vi "user process.vi"(8 "error in":errorcluster, 10 "MotionModule runtime in":refnum<class "MotionModule runtime.lvclass">, 11 "Parameters to process":T2) -> (0 "error out":errorcluster, 2 "MotionModule runtime Out":refnum<class "MotionModule runtime.lvclass">, 3 "Results from processing":T1)   [LabVIEW 2017, in "MotionModule runtime.lvclass"]
uses:
  MotionModule runtime.lvclass
  parameter user data.ctl
  result user data.ctl
  MotionModule runtime.lvclass/MotionModule runtime.ctl
  Utilities/StateMachine.ctl
  SoftmotionClass/SoftmotionAxis/SoftmotionAxis.lvclass
  Utilities/Controlword_Commands.ctl
  Utilities/MoveMode.ctl
  Utilities/WordManipulationLibrary.lvlib
  Utilities/Bit Manipulation.lvlib
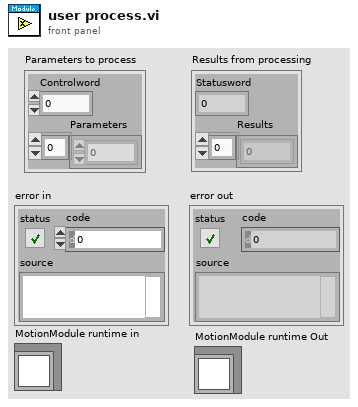
[diagram p1: front panel]
types:
  T1 = typedef "MotionModule runtime.lvclass/result user data.ctl" = cluster{"Statusword":u16, "Results":dbl[]}
  T2 = typedef "MotionModule runtime.lvclass/parameter user data.ctl" = cluster{"Controlword":u16, "Parameters":dbl[]}
  T3 = typedef "WordManipulationLibrary.lvlib/StateMachine.ctl" = enum16{"Start", "Not Ready to Switch On", "Switch On Disabled", "Ready to Switch On", "Switched On", "Operation enable", "Quick Stop Active", "Fault Reaction Active", "Fault"}
  T4 = typedef "WordManipulationLibrary.lvlib/Controlword_Commands.ctl" = enum16{"Shutdown", "Switch On", "Disable Voltage", "Quick Stop", "Disable Op", "Enable Op", "Fault Reset", "Error"}
  T5 = typedef "WordManipulationLibrary.lvlib/MoveMode.ctl" = enum16{"Reserved", "Profile Position Mode", "Velocity Mode", "Profile Velocity Mode", "Profile Torque Mode", "Reserved 2", "Reference Mode", "Interpolated Position Mode", "Skip"}
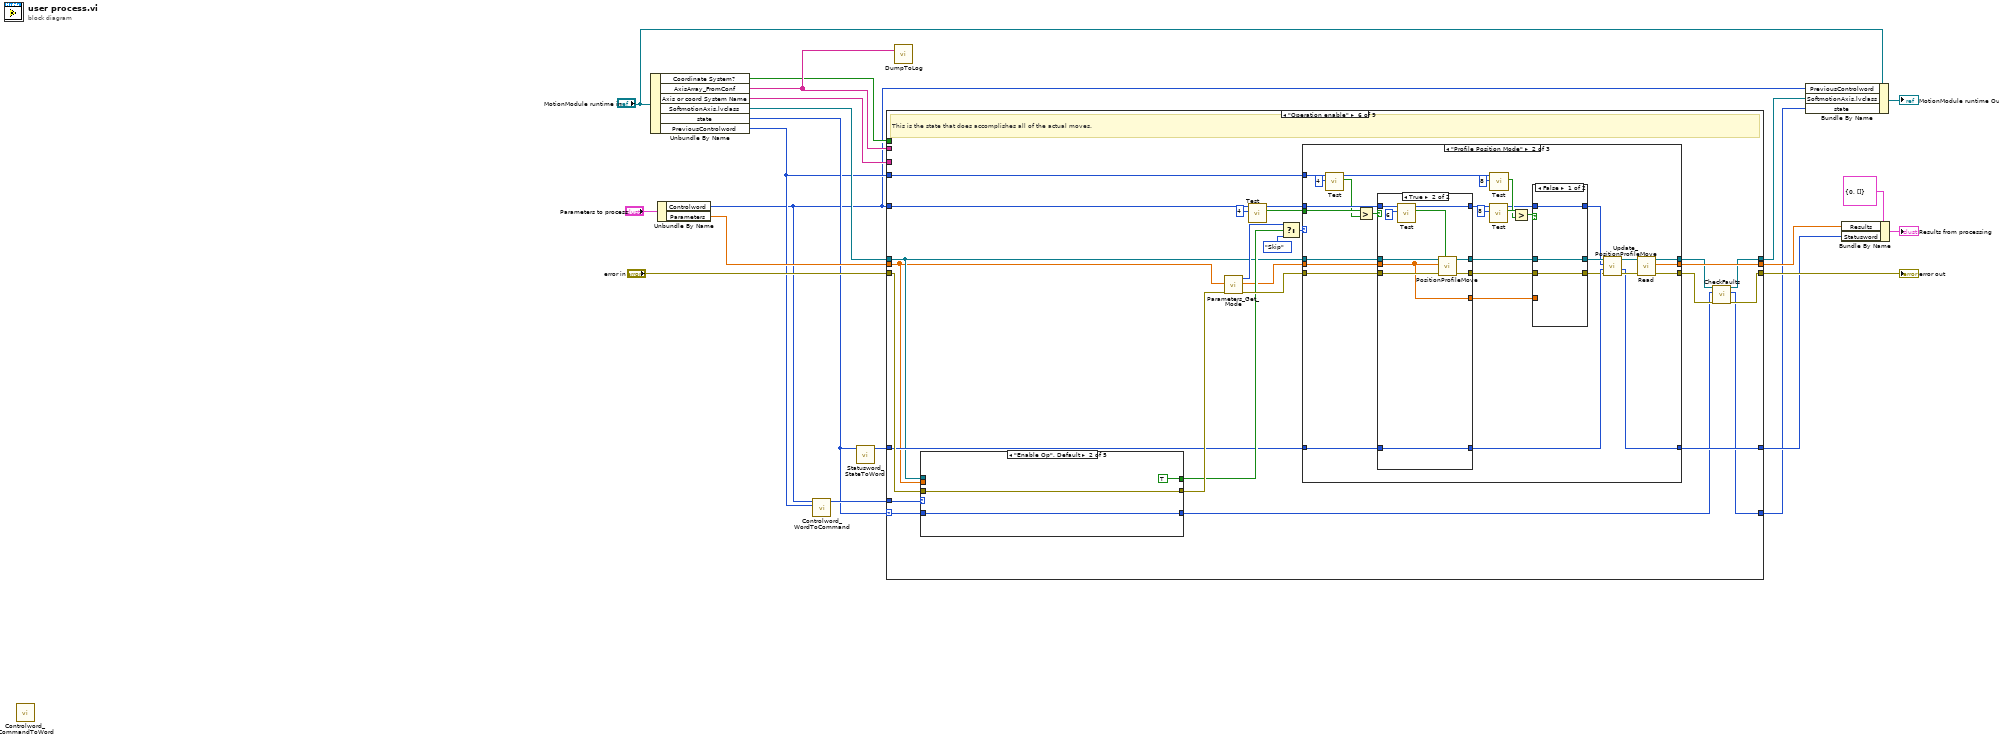
[diagram p0: block diagram]
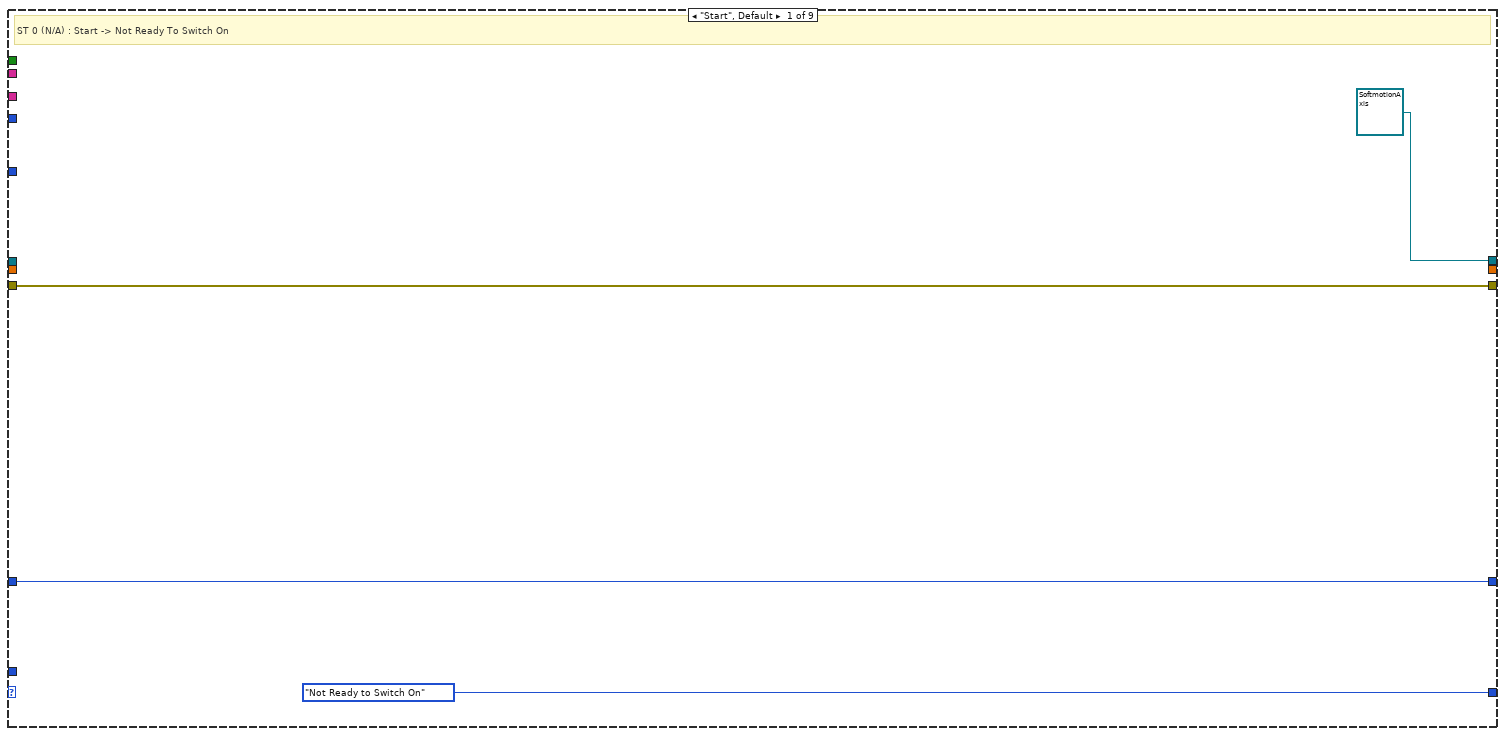
[diagram p2: hidden frame]
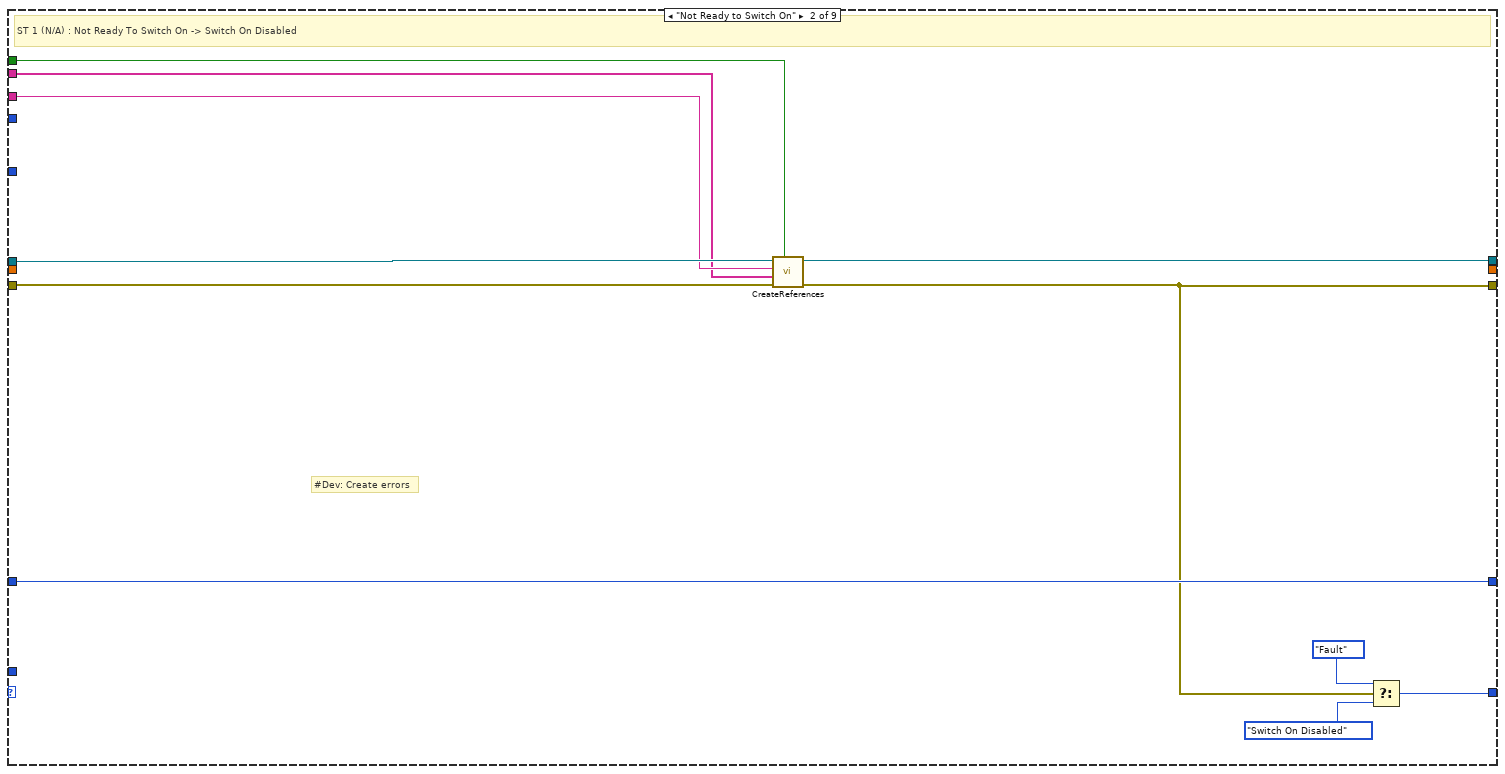
[diagram p3: hidden frame]
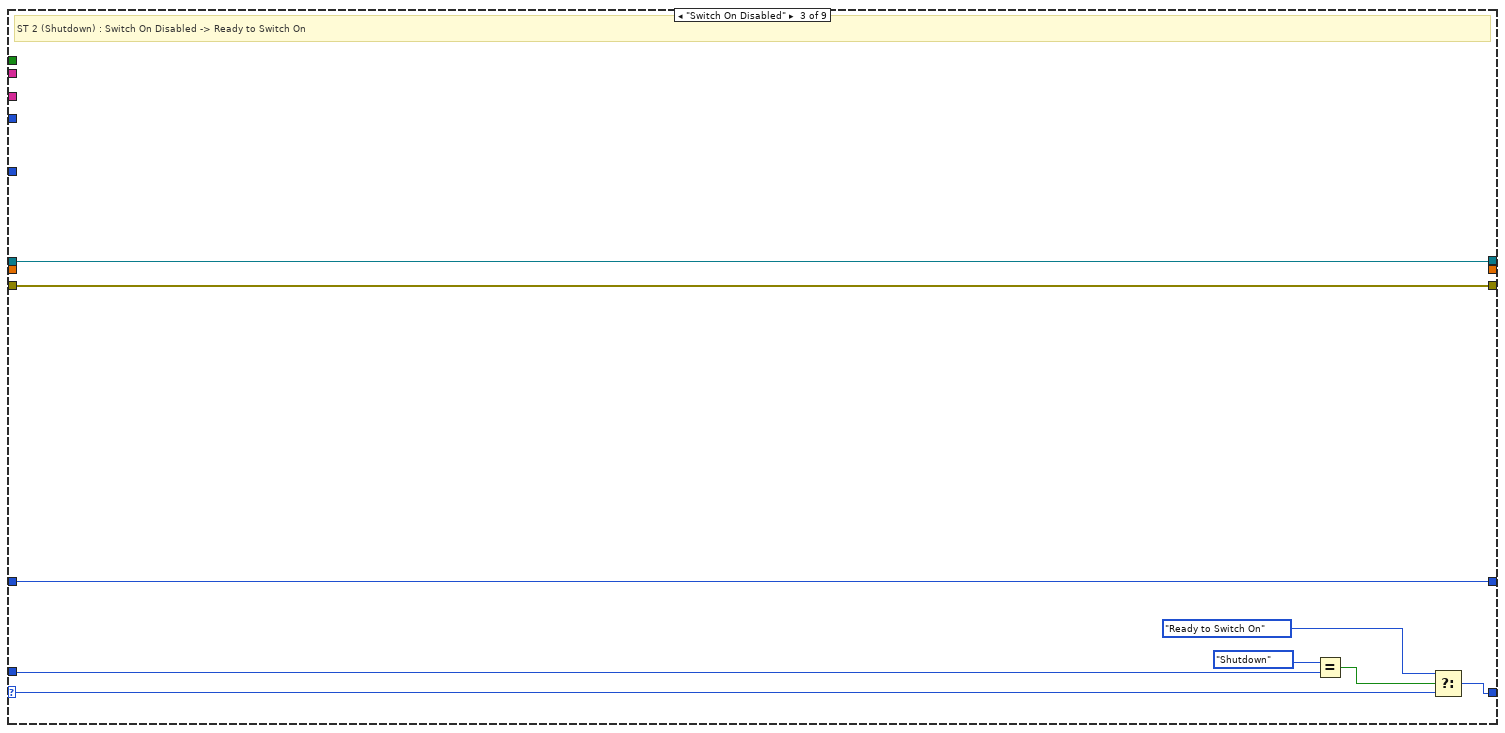
[diagram p4: hidden frame]
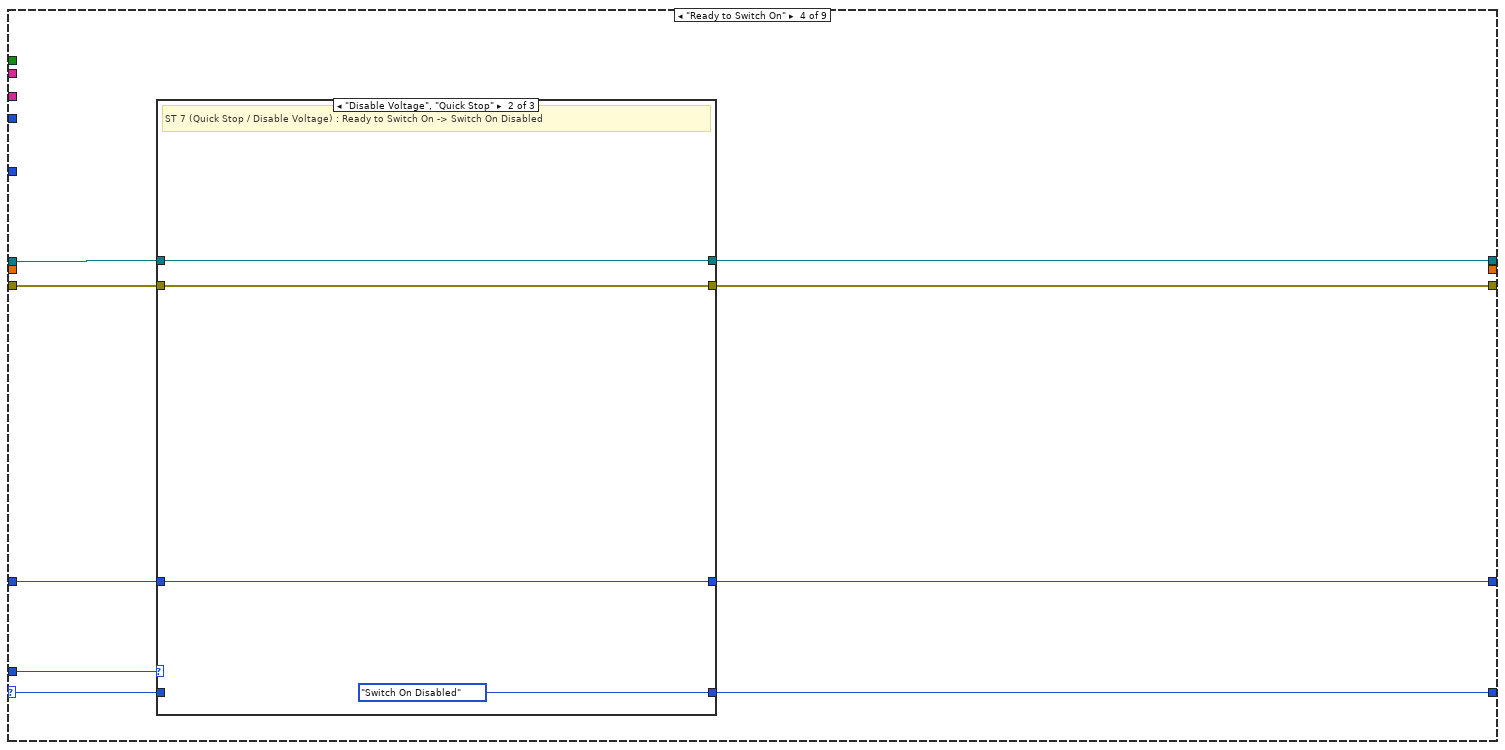
[diagram p5: hidden frame]
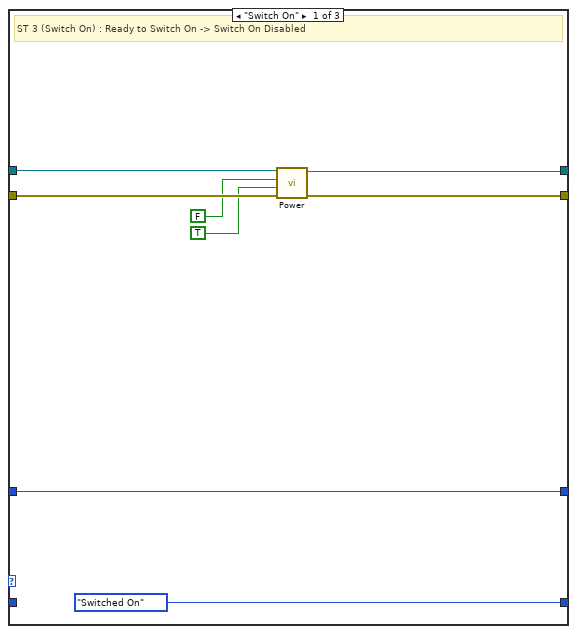
[diagram p6: hidden frame]
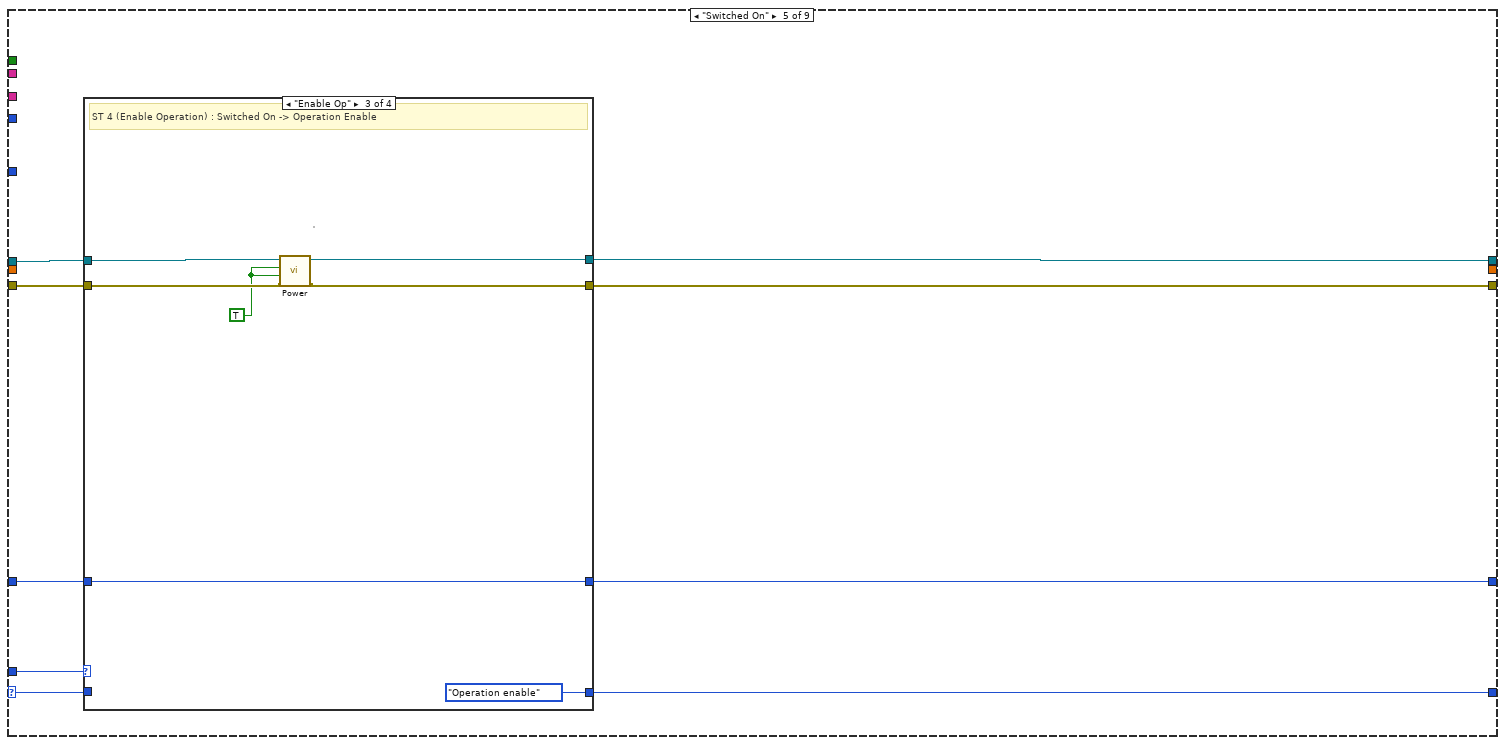
[diagram p8: hidden frame]
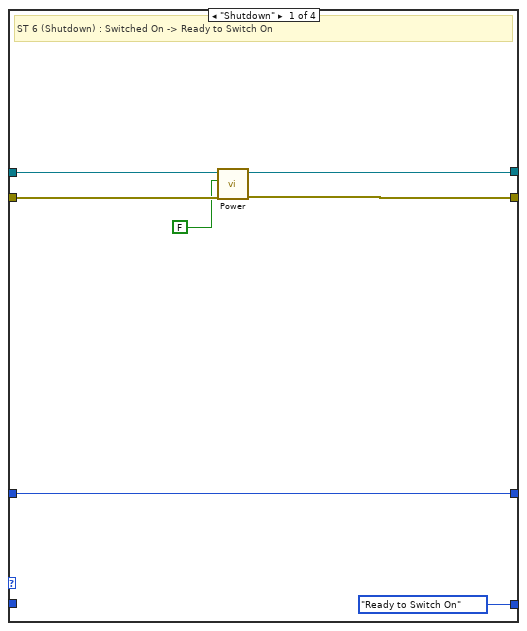
[diagram p9: hidden frame]
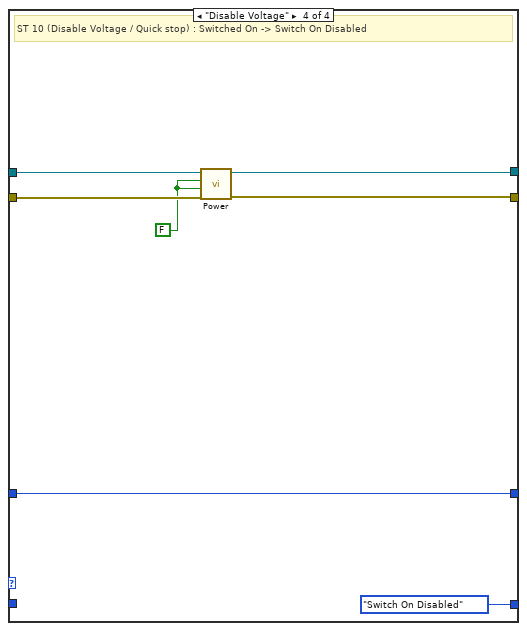
[diagram p11: hidden frame]
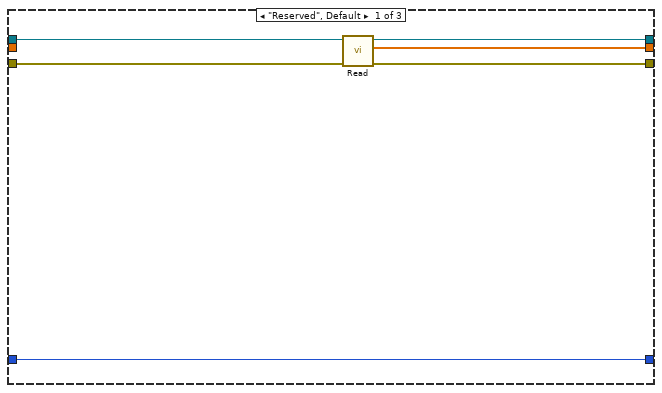
[diagram p12: hidden frame]
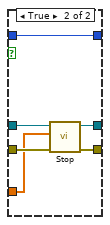
[diagram p13: hidden frame]
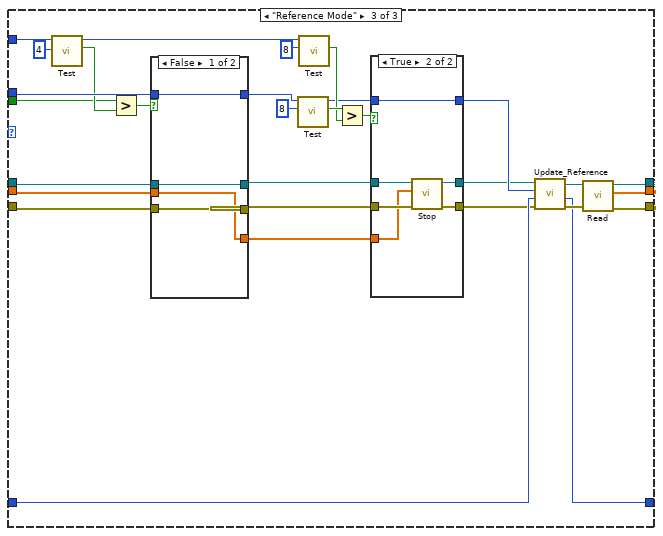
[diagram p15: hidden frame]
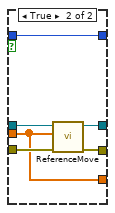
[diagram p17: hidden frame]
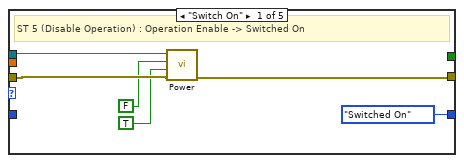
[diagram p18: hidden frame]
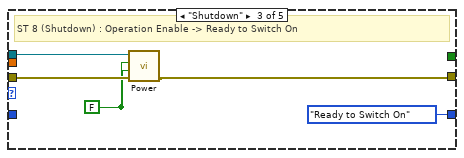
[diagram p19: hidden frame]
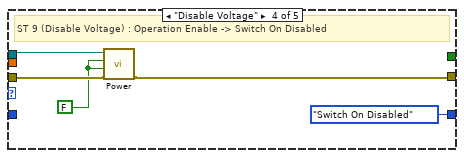
[diagram p20: hidden frame]
diagram:
  n1 = call "Controlword_CommandToWord.vi"() -> ()  [unwired: 11 in, 1 out]
  n2 = Unbundle By Name("MotionModule runtime in") -> ("Coordinate System?"=w2:bool, "AxisArray_FromConf"=w3:string[], "Axis or coord System Name"=w5:string, "SoftmotionAxis.lvclass"=w15:refnum<class "SoftmotionAxis.lvclass">, "state"=w7:T3, "PreviousControlword"=w4:u16)
  n3 = Unbundle By Name("Parameters to process") -> ("Controlword"=w1:u16, "Parameters"=w18:dbl[])
  n4 = call "Controlword_WordToCommand.vi"("Previous Controlword"=w4, "Controlword"=w1) -> ("Device Control Command"=w20:T4)  [unwired: 9 in]
  n5 = call "Statusword_StateToWord.vi"("CurrentStatus"=w7) -> ("StatusWord Out"=w21:u16)  [unwired: 10 in]
  n6 = case shown="\"Operation enable\"" w7 {
    selector: w7 -> [_ _ w41 w53 w78 w129 w267 _ w285]
    tunnel: w20 -> [_ _ w45 w54 w79 w130 w269 _ w286]
    tunnel: [StateMachine."Not Ready to Switch On" w33 w40 w52 w77 w107 w268 StateMachine."Fault" w287] -> w6
    tunnel: [w24 w36 w39 w48 w74 w126 w266 w278 w284] -> w8
    tunnel: w21 -> [w24 w36 w39 w49 w75 w115 w266 w278 w284]
    tunnel: w1 -> [_ _ _ _ _ w128 _ _ _]
    tunnel: w18 -> [_ _ _ _ _ w105 _ _ _]
    tunnel: w5 -> [_ w28 _ _ _ _ _ _ _]
    tunnel: [_ _ _ _ _ w125 _ _ _] -> w9
    tunnel: "error in" -> [w23 w32 w38 w51 w76 w121 _ w275 w283]
    tunnel: [w23 w29 w38 w50 w73 w111 _ w274 w282] -> w16
    tunnel: w15 -> [_ w31 w37 w47 w72 w113 w265 w277 w281]
    tunnel: [refnum<class "SoftmotionAxis.lvclass"> refnum ("SoftmotionAxis.lvclass") w30 w37 w46 w71 w109 w265 w276 w280] -> w13
    tunnel: w4 -> [_ _ _ _ _ w106 _ _ _]
    tunnel: w3 -> [_ w26 _ _ _ _ _ _ _]
    tunnel: w2 -> [_ w27 _ _ _ _ _ _ _]
    frame "Start", Default {
      # "ST 0 (N/A) : Start -> Not Ready To Switch On"
    }
    frame "Not Ready to Switch On" {
      # "#Dev: Create errors"
      # "ST 1 (N/A) : Not Ready To Switch On -> Switch On Disabled"
      n7 = call-dynamic "CreateReferences.vi"("Coorinate System?"=w27, "error in (no error)"=w32, "AxisArray_FromConf"=w26, "Axis Name"=w28, "SoftmotionAxis in"=w31) -> ("error out"=w29:errorcluster, "SoftmotionAxis out"=w30:refnum<class "SoftmotionAxis.lvclass">)  [unwired: 5 in]
      n8 = Select(t=StateMachine."Fault", s=w29, f=StateMachine."Switch On Disabled") -> (s? t:f=w33:T3)
    }
    frame "Switch On Disabled" {
      # "ST 2 (Shutdown) : Switch On Disabled -> Ready to Switch On"
      n9 = Equal?(x=Controlword_Commands."Shutdown" ("Device Control Command"), y=w45) -> (x = y?=w44:bool)
      n10 = Select(t=StateMachine."Ready to Switch On", s=w44, f=w41) -> (s? t:f=w40:T3)
    }
    frame "Ready to Switch On" {
      n11 = case shown="\"Disable Voltage\", \"Quick Stop\"" w54 {
        tunnel: w53 -> [_ _ w70]
        tunnel: [StateMachine."Switched On" StateMachine."Switch On Disabled" w70] -> w52
        tunnel: w51 -> [w59 w65 w69]
        tunnel: [w60 w65 w69] -> w50
        tunnel: [w61 w64 w68] -> w48
        tunnel: w49 -> [w61 w64 w68]
        tunnel: w47 -> [w58 w63 w67]
        tunnel: [w55 w63 w67] -> w46
        frame "Switch On" {
          # "ST 3 (Switch On) : Ready to Switch On -> Switch On Disabled"
          n12 = call-dynamic "Power.vi"("error in (no error)"=w59, "Enable Drive"=TRUE, "Enable Axis"=FALSE, "SoftmotionAxis in"=w58) -> ("error out"=w60:errorcluster, "SoftmotionAxis out"=w55:refnum<class "SoftmotionAxis.lvclass">)  [unwired: 6 in]
        }
        frame "Disable Voltage", "Quick Stop" {
          # "ST 7 (Quick Stop / Disable Voltage) : Ready to Switch On -> Switch On Disabled"
        }
        frame Default {
          # "No Op."
        }
      }
    }
    frame "Switched On" {
      n13 = case shown="\"Enable Op\"" w79 {
        tunnel: w78 -> [_ w90 _ _]
        tunnel: [StateMachine."Ready to Switch On" w90 StateMachine."Operation enable" StateMachine."Switch On Disabled"] -> w77
        tunnel: w76 -> [w84 w89 w95 w102]
        tunnel: [w83 w89 w94 w101] -> w73
        tunnel: [w85 w88 w96 w103] -> w74
        tunnel: w75 -> [w85 w88 w96 w103]
        tunnel: w72 -> [w81 w87 w93 w100]
        tunnel: [w80 w87 w91 w99] -> w71
        frame "Shutdown" {
          # "ST 6 (Shutdown) : Switched On -> Ready to Switch On"
          n14 = call-dynamic "Power.vi"("error in (no error)"=w84, "Enable Axis"=FALSE, "SoftmotionAxis in"=w81) -> ("error out"=w83:errorcluster, "SoftmotionAxis out"=w80:refnum<class "SoftmotionAxis.lvclass">)  [unwired: 7 in]
        }
        frame Default {
          # "No op"
        }
        frame "Enable Op" {
          w92 = TRUE ("Enable Axis")
          # "ST 4 (Enable Operation) : Switched On -> Operation Enable"
          n15 = call-dynamic "Power.vi"("error in (no error)"=w95, "Enable Drive"=w92, "Enable Axis"=w92, "SoftmotionAxis in"=w93) -> ("error out"=w94:errorcluster, "SoftmotionAxis out"=w91:refnum<class "SoftmotionAxis.lvclass">)  [unwired: 6 in]
        }
        frame "Disable Voltage" {
          w98 = FALSE ("Enable Axis")
          # "ST 10 (Disable Voltage / Quick stop) : Switched On -> Switch On Disabled"
          n16 = call-dynamic "Power.vi"("error in (no error)"=w102, "Enable Drive"=w98, "Enable Axis"=w98, "SoftmotionAxis in"=w100) -> ("error out"=w101:errorcluster, "SoftmotionAxis out"=w99:refnum<class "SoftmotionAxis.lvclass">)  [unwired: 6 in]
        }
      }
    }
    frame "Operation enable" {
      # "This is the state that does accomplishes all of the actual moves."
      n17 = case shown="\"Enable Op\", Default" w130 {
        tunnel: w129 -> [_ w249 _ _ _]
        tunnel: [StateMachine."Switched On" w249 StateMachine."Ready to Switch On" StateMachine."Switch On Disabled" StateMachine."Quick Stop Active"] -> w108
        tunnel: w121 -> [w245 w248 w253 w258 w263]
        tunnel: [w244 w248 w252 w257 w262] -> w120
        tunnel: [_ TRUE _ _ _] -> w117
        tunnel: w113 -> [w243 _ w250 w255 w261]
        tunnel: w105 -> [_ _ _ _ w260]
        frame "Switch On" {
          # "ST 5 (Disable Operation) : Operation Enable -> Switched On"
          n18 = call-dynamic "Power.vi"("error in (no error)"=w245, "Enable Drive"=TRUE, "Enable Axis"=FALSE, "SoftmotionAxis in"=w243) -> ("error out"=w244:errorcluster)  [unwired: 6 in, 1 out]
        }
        frame "Enable Op", Default {
        }
        frame "Shutdown" {
          w251 = FALSE ("Enable Axis")
          # "ST 8 (Shutdown) : Operation Enable -> Ready to Switch On"
          n19 = call-dynamic "Power.vi"("error in (no error)"=w253, "Enable Drive"=w251, "Enable Axis"=w251, "SoftmotionAxis in"=w250) -> ("error out"=w252:errorcluster)  [unwired: 6 in, 1 out]
        }
        frame "Disable Voltage" {
          w256 = FALSE ("Enable Axis")
          # "ST 9 (Disable Voltage) : Operation Enable -> Switch On Disabled"
          n20 = call-dynamic "Power.vi"("error in (no error)"=w258, "Enable Drive"=w256, "Enable Axis"=w256, "SoftmotionAxis in"=w255) -> ("error out"=w257:errorcluster)  [unwired: 6 in, 1 out]
        }
        frame "Quick Stop" {
          # "ST 11 (Quick Stop) : Operation Enable -> Quick Stop Active"
          n21 = call-dynamic "Stop.vi"("error in (no error)"=w263, "Parameters"=w260, "SoftmotionAxis in"=w261) -> ("error out"=w262:errorcluster)  [unwired: 7 in, 1 out]
        }
      }
      n22 = call "Parameters_Get_Mode.vi"("error in (no error)"=w120, "Parameters"=w105) -> ("error out"=w122:errorcluster, "Parameters Out"=w114:dbl[], "Move Mode"=w119:T5)  [unwired: 7 in]
      n23 = call "Test.vi"("Bit to test"=u8 4, "Data_In"=w128) -> ("bit value"=w123:bool, "Data_Out"=w124:u16)  [unwired: 8 in]
      n24 = Select(t=w119, s=w117, f=MoveMode."Skip") -> (s? t:f=w118:T5)
      n25 = case shown="\"Profile Position Mode\"" w118 {
        tunnel: w123 -> [_ w164 w207]
        tunnel: [w136 w154 w211] -> w126
        tunnel: w115 -> [w136 w162 w212]
        tunnel: [w135 w160 w217] -> w125
        tunnel: w124 -> [_ w167 w215]
        tunnel: w114 -> [_ w165 w220]
        tunnel: w122 -> [w133 w166 w219]
        tunnel: [w134 w159 w218] -> w112
        tunnel: w113 -> [w132 w161 w221]
        tunnel: [w131 w158 w216] -> w110
        tunnel: w106 -> [_ w152 w208]
        frame "Reserved", Default {
          n26 = call-dynamic "Read.vi"("error in (no error)"=w133, "SoftmotionAxis in"=w132) -> ("error out"=w134:errorcluster, "appended array"=w135:dbl[], "SoftmotionAxis out"=w131:refnum<class "SoftmotionAxis.lvclass">)  [unwired: 7 in]
        }
        frame "Profile Position Mode" {
          n27 = call "Test.vi"("Bit to test"=u8 4, "Data_In"=w152) -> ("bit value"=w151:bool, "Data_Out"=w142:u16)  [unwired: 8 in]
          n28 = Greater?(x=w164, y=w151) -> (0:w163:bool)
          n29 = case shown="True" w163 {
            tunnel: w167 -> [w181 w191]
            tunnel: w166 -> [w179 w189]
            tunnel: w165 -> [w177 w182]
            tunnel: w162 -> [w178 w183]
            tunnel: w161 -> [w180 w187]
            tunnel: [w180 w186] -> w146
            tunnel: [w179 w185] -> w149
            tunnel: [w181 w184] -> w150
            tunnel: [w178 w183] -> w155
            tunnel: [w177 w182] -> w137
            frame False {
            }
            frame True {
              n30 = call "Test.vi"("Bit to test"=u8 6, "Data_In"=w191) -> ("bit value"=w188:bool, "Data_Out"=w184:u16)  [unwired: 8 in]
              n31 = call-dynamic "PositionProfileMove.vi"("Relative?"=w188, "error in (no error)"=w189, "Array"=w182, "SoftmotionAxis in"=w187) -> ("error out"=w185:errorcluster, "SoftmotionAxis out"=w186:refnum<class "SoftmotionAxis.lvclass">)  [unwired: 6 in]
            }
          }
          n32 = call "Test.vi"("Bit to test"=u8 8, "Data_In"=w150) -> ("bit value"=w144:bool, "Data_Out"=w139:u16)  [unwired: 8 in]
          n33 = call "Test.vi"("Bit to test"=u8 8, "Data_In"=w142) -> ("bit value"=w141:bool)  [unwired: 8 in, 1 out]
          n34 = Greater?(x=w144, y=w141) -> (0:w140:bool)
          n35 = case shown="False" w140 {
            tunnel: w149 -> [w170 w176]
            tunnel: [w170 w175] -> w148
            tunnel: [w169 w174] -> w147
            tunnel: w146 -> [w169 w173]
            tunnel: w139 -> [w168 w172]
            tunnel: [w168 w172] -> w138
            tunnel: w137 -> [_ w171]
            frame False {
            }
            frame True {
              n36 = call-dynamic "Stop.vi"("error in (no error)"=w176, "Parameters"=w171, "SoftmotionAxis in"=w173) -> ("error out"=w175:errorcluster, "SoftmotionAxis out"=w174:refnum<class "SoftmotionAxis.lvclass">)  [unwired: 7 in]
            }
          }
          n37 = call-dynamic "Update_PositionProfileMove.vi"("error in (no error)"=w148, "StatusWord"=w155, "ControlWord"=w138, "SoftmotionAxis in"=w147) -> ("error out"=w156:errorcluster, "StatusWord Out"=w154:u16, "SoftmotionAxis out"=w157:refnum<class "SoftmotionAxis.lvclass">)  [unwired: 5 in]
          n38 = call-dynamic "Read.vi"("error in (no error)"=w156, "SoftmotionAxis in"=w157) -> ("error out"=w159:errorcluster, "appended array"=w160:dbl[], "SoftmotionAxis out"=w158:refnum<class "SoftmotionAxis.lvclass">)  [unwired: 7 in]
        }
        frame "Reference Mode" {
          n39 = call "Test.vi"("Bit to test"=u8 4, "Data_In"=w208) -> ("bit value"=w210:bool, "Data_Out"=w199:u16)  [unwired: 8 in]
          n40 = Greater?(x=w207, y=w210) -> (0:w206:bool)
          n41 = case shown="False" w206 {
            tunnel: w215 -> [w232 w236]
            tunnel: w219 -> [w234 w240]
            tunnel: w220 -> [w231 w235]
            tunnel: [w234 w237] -> w193
            tunnel: w221 -> [w233 w239]
            tunnel: [w233 w238] -> w194
            tunnel: [w232 w236] -> w198
            tunnel: [w231 w235] -> w192
            frame False {
            }
            frame True {
              n42 = call-dynamic "ReferenceMove.vi"("error in (no error)"=w240, "Array"=w235, "SoftmotionAxis in"=w239) -> ("error out"=w237:errorcluster, "SoftmotionAxis out"=w238:refnum<class "SoftmotionAxis.lvclass">)  [unwired: 7 in]
            }
          }
          n43 = call "Test.vi"("Bit to test"=u8 8, "Data_In"=w198) -> ("bit value"=w204:bool, "Data_Out"=w200:u16)  [unwired: 8 in]
          n44 = call "Test.vi"("Bit to test"=u8 8, "Data_In"=w199) -> ("bit value"=w202:bool)  [unwired: 8 in, 1 out]
          n45 = Greater?(x=w204, y=w202) -> (0:w201:bool)
          n46 = case shown="True" w201 {
            tunnel: w193 -> [w224 w230]
            tunnel: [w224 w229] -> w195
            tunnel: [w223 w228] -> w196
            tunnel: w194 -> [w223 w227]
            tunnel: w200 -> [w222 w226]
            tunnel: [w222 w226] -> w197
            tunnel: w192 -> [_ w225]
            frame False {
            }
            frame True {
              n47 = call-dynamic "Stop.vi"("error in (no error)"=w230, "Parameters"=w225, "SoftmotionAxis in"=w227) -> ("error out"=w229:errorcluster, "SoftmotionAxis out"=w228:refnum<class "SoftmotionAxis.lvclass">)  [unwired: 7 in]
            }
          }
          n48 = call "Update_Reference.vi"("error in (no error)"=w195, "StatusWord"=w212, "ControlWord"=w197, "SoftmotionAxis in"=w196) -> ("error out"=w214:errorcluster, "StatusWord Out"=w211:u16, "SoftmotionAxis out"=w213:refnum<class "SoftmotionAxis.lvclass">)  [unwired: 5 in]
          n49 = call-dynamic "Read.vi"("error in (no error)"=w214, "SoftmotionAxis in"=w213) -> ("error out"=w218:errorcluster, "appended array"=w217:dbl[], "SoftmotionAxis out"=w216:refnum<class "SoftmotionAxis.lvclass">)  [unwired: 7 in]
        }
      }
      n50 = call "CheckFaults.vi"("error in (no error)"=w112, "State In"=w108, "SoftmotionAxis in"=w110) -> ("error out"=w111:errorcluster, "State Out"=w107:T3, "SoftmotionAxis out"=w109:refnum<class "SoftmotionAxis.lvclass">)  [unwired: 6 in]
    }
    frame "Quick Stop Active" {
      # "#Dev: If the Quick Stop action ends, then the system goes to Switch On Disable as well."
      n51 = case shown="\"Shutdown\", Default" w269 {
        tunnel: w267 -> [_ _ w272]
        tunnel: [StateMachine."Operation enable" StateMachine."Switch On Disabled" w272] -> w268
        frame "Enable Op" {
          # "ST 16 (Enable Operation) : Quick Stop Active -> Operation Enable"
        }
        frame "Disable Voltage" {
          # "ST 12 (Quick Stop / Disable Voltage) : Quick Stop Active -> Switch On Disabled"
        }
        frame "Shutdown", Default {
          # "No Transition"
        }
      }
    }
    frame "Fault Reaction Active" {
      w273 = FALSE ("Enable Axis")
      # "#Dev: Deal with Fault here (Log, communicate, etc)"
      # "ST 14 (N/A) : Fault Reaction Active -> Fault"
      n52 = call-dynamic "Power.vi"("error in (no error)"=w275, "Enable Drive"=w273, "Enable Axis"=w273, "SoftmotionAxis in"=w277) -> ("error out"=w274:errorcluster, "SoftmotionAxis out"=w276:refnum<class "SoftmotionAxis.lvclass">)  [unwired: 6 in]
    }
    frame "Fault" {
      n53 = case shown="\"Shutdown\", Default" w286 {
        tunnel: [w290 StateMachine."Switch On Disabled"] -> w287
        tunnel: w285 -> [w290 _]
        tunnel: w281 -> [w288 w294]
        tunnel: w283 -> [w289 w293]
        tunnel: [w289 w292] -> w282
        tunnel: [w288 w291] -> w280
        frame "Shutdown", Default {
        }
        frame "Fault Reset" {
          n54 = call-dynamic "ClearFaults.vi"("error in (no error)"=w293, "SoftmotionAxis in"=w294) -> ("error out"=w292:errorcluster, "SoftmotionAxis out"=w291:refnum<class "SoftmotionAxis.lvclass">)  [unwired: 8 in]
        }
      }
    }
  }
  "error out" <- w16
  n55 = call "DumpToLog.vi"("DataToLog"=w3) -> ()  [unwired: 11 in]
  n56 = Bundle By Name(cluster="MotionModule runtime in", "PreviousControlword"=w1, "SoftmotionAxis.lvclass"=w13, "state"=w6) -> (→"MotionModule runtime Out":refnum<class "MotionModule runtime.lvclass">)
  n57 = Bundle By Name(cluster=T1 {"Statusword"=0, "Results"=[]} ("Results from processing"), "Results"=w9, "Statusword"=w8) -> (→"Results from processing":T1)
